vi "Find baseplate center.vi"() -> ()   [LabVIEW 2020]
uses:
  Classes/Workspace/Workspace.ctl
  Classes/Workspace/Carrier Tray/Assembly Tray.lvclass
  Classes/Controller/Controller.lvclass
  Classes/Workspace/Fixture.lvclass
panel:
  out "Workspace":T1
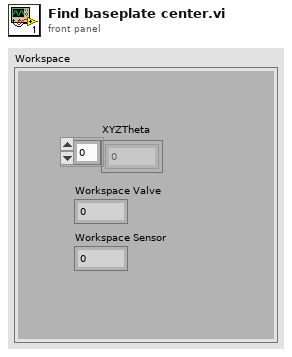
[diagram p1: front panel]
types:
  T1 = typedef "Fixture.lvclass/Workspace.ctl" = cluster{"XYZTheta":dbl[], "Workspace Valve":i32, "Workspace Sensor":i32}
  T2 = typedef "Controller.lvclass/Controllers.ctl" = cluster{"I-O.lvclass":refnum<class "I-O.lvclass">, "Dispenser.lvclass":refnum<class "Dispenser.lvclass">, "Gantry":refnum<k24>}
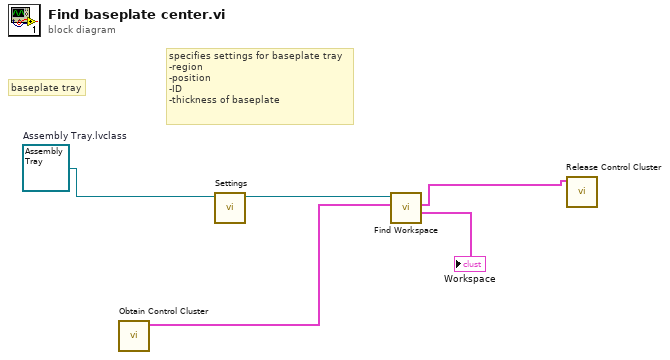
[diagram p0: block diagram]
diagram:
  w5 = refnum<class "Assembly Tray.lvclass"> refnum  # Assembly Tray.lvclass
  # "specifies settings for baseplate tray\n-region\n-position\n-ID \n-thickness of baseplate"
  # "baseplate tray"
  n1 = call "Obtain Control Cluster.vi"() -> ("Control Out"=w3:T2)  [unwired: 11 in]
  n2 = call-dynamic "Settings.vi"("Assembly Tray In"=w5) -> ("Assembly Tray Out"=w4:refnum<class "Assembly Tray.lvclass">)  [unwired: 9 in, 1 out]
  n3 = call-dynamic "Find Workspace.vi"("Control In"=w3, "Carrier Tray in"=w4) -> ("Workspace"=→"Workspace":T1, "Control Out"=w2:T2)  [unwired: 6 in, 2 out]
  n4 = call "Release Control Cluster.vi"("output cluster"=w2) -> ()  [unwired: 11 in]
